vi "AlliGator Supported FLI Dataset Files.vi"() -> (5 "Pattern String":string, 7 "File Extensions":string[](array[string]))   [LabVIEW 2021, in "AlliGator Files.lvlib"]
doc: "Returns a string of supported image file name patterns that can be used in a File Dialog (*.hdf5; *.ptu; etc. and their uppercase variants) and an array of the same extensions (without the \"*\" or \".\" characters)."
uses:
  AlliGator Files.lvlib
panel:
  # "see the AlliGator License on the block diagram (Ctrl+E or Window:Show Block Diagram)"
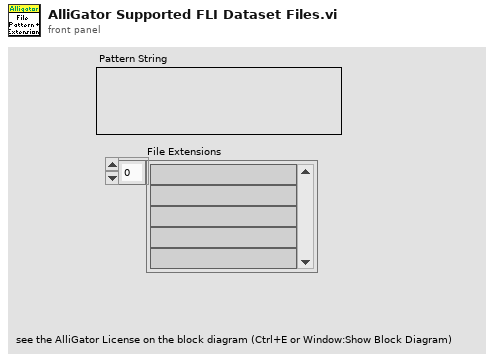
[diagram p1: front panel]
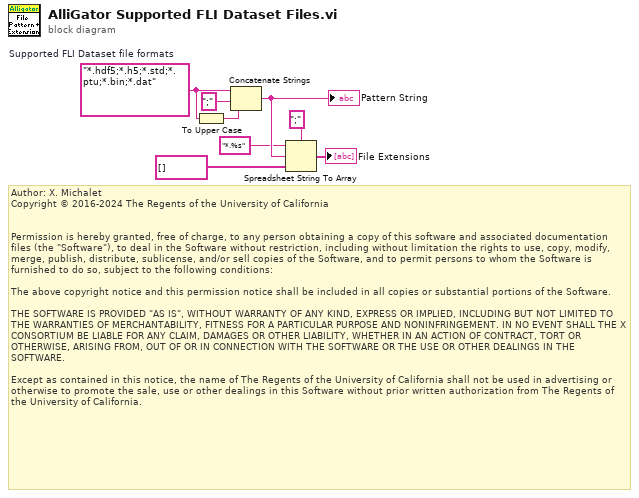
[diagram p0: block diagram]
diagram:
  w7 = "*.hdf5;*.h5;*.std;*.ptu;*.bin;*.dat"  # Supported FLI Dataset file formats
  # "Author: X. Michalet\nCopyright © 2016-2024 The Regents of the University of California\n \n\nPermission is hereby granted, free of charge, to any person obtaining a copy of this software and associated documentation files (the \"Software\"), to deal in the Software without restriction, including without limitation the rights to use, copy, modify, merge, publish, distribute, sublicense, and/or sell copies of the Software, and to permit persons to whom the Software is furnished to do so, subject to the following conditions:\n\nThe above copyright notice and this permission notice shall be included in all copies or substantial portions of the Software.\n\nTHE SOFTWARE IS PROVIDED \"AS IS\", WITHOUT WARRANTY OF ANY KIND, EXPRESS OR IMPLIED, INCLUDING BUT NOT LIMITED TO THE WARRANTIES OF MERCHANTABILITY, FITNESS FOR A PARTICULAR PURPOSE AND NONINFRINGEMENT. IN NO EVENT SHALL THE X CONSORTIUM BE LIABLE FOR ANY CLAIM, DAMAGES OR OTHER LIABILITY, WHETHER IN AN ACTION OF CONTRACT, TORT OR OTHERWISE, ARISING FROM, OUT OF OR IN CONNECTION WITH THE SOFTWARE OR THE USE OR OTHER DEALINGS IN THE SOFTWARE.\n\nExcept as contained in this notice, the name of The Regents of the University of California shall not be used in advertising or otherwise to promote the sale, use or other dealings in this Software without prior written authorization from The Regents of the University of California."
  n1 = To Upper Case(1:w7) -> (0:w8:string)
  n2 = Concatenate Strings(w7, ";" ("string"), w8) -> (w5:string)
  "Pattern String" <- w5
  n3 = Spreadsheet String To Array(delimiter (Tab)=";", format string="*.%s", spreadsheet string=w5, array type (2D Dbl)=string[] []) -> (array=→"File Extensions":string[])
